vi "Img_PreProcess.vi"(4 "copy_name":string="untitled", 6 "copy_img":bool, 8 "error in (no error)":errorcluster, 11 "Original Img":T1) -> (0 "error out":errorcluster, 2 "transformed_out":T1, 3 "Original Img out":T1)   [LabVIEW 2021, in "Framework_lib.lvlib"]
uses:
  QMH/Framework_lib.lvlib
  <vilib>/vision/Image Controls.llb/IMAQ Image.ctl
  <vilib>/vision/NI_Vision_Development_Module.lvlib
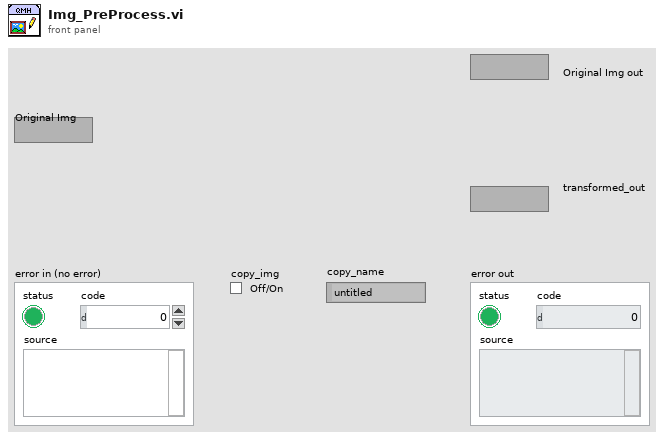
[diagram p1: front panel]
types:
  T1 = typedef "IMAQ Image.ctl" = refnum<image>
  T2 = cluster{"Brightness":sgl, "Contrast":sgl, "Gamma":sgl}
  T3 = typedef "Image Type" = u32
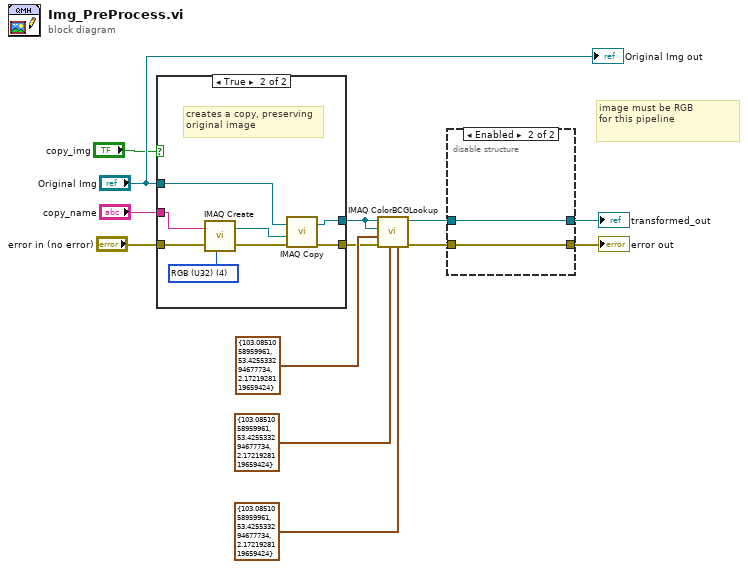
[diagram p0: block diagram]
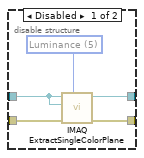
[diagram p2: hidden frame]
diagram:
  # "image must be RGB\nfor this pipeline"
  n1 = case shown="True" "copy_img" {
    tunnel: "error in (no error)" -> [w15 w23]
    tunnel: [w15 w22] -> w6
    tunnel: "Original Img" -> [w14 w21]
    tunnel: [w14 w20] -> w1
    tunnel: "copy_name" -> [_ w18]
    frame False {
      # "will transform orignial image"
    }
    frame True {
      w17 = T3 4 items=["Grayscale (U8)", "Grayscale (I16)", "Grayscale (SGL)", "Complex (CSG)", "RGB (U32)", "HSL (U32)", "RGB (U64)", "Grayscale (U16)"] ("Image Type")
      # "creates a copy, preserving\noriginal image"
      n2 = call "IMAQ Create"("Image Name"=w18, "Image Type"=w17, "error in (no error)"=w23) -> ("New Image"=w16:T1, "error out"=w19:errorcluster)  [unwired: 2 in]
      n3 = call "IMAQ Copy"("error in (no error)"=w19, "Image Dst"=w16, "Image Src"=w21) -> ("error out"=w22:errorcluster, "Image Dst Out"=w20:T1)  [unwired: 3 in]
    }
  }
  n4 = call "IMAQ ColorBCGLookup"("Blue BCG Values"=T2 {"Brightness"=103.085106, "Contrast"=53.425533, "Gamma"=2.1721928}, "Green BCG Values"=T2 {"Brightness"=103.085106, "Contrast"=53.425533, "Gamma"=2.1721928}, "error in (no error)"=w6, "Red BCG Values"=T2 {"Brightness"=103.085106, "Contrast"=53.425533, "Gamma"=2.1721928}, "Image Dst"=w1, "Image Src"=w1) -> ("error out"=w8:errorcluster, "Image Dst Out"=w3:T1)  [unwired: 1 in, 3 out]
  n5 = disable-structure shown="Enabled" {
    disable-tunnel: [w28 w29] -> w13
    disable-tunnel: [w27 w30] -> w12
    disable-tunnel: w8 -> [w25 w30]
    disable-tunnel: w3 -> [w24 w29]
    frame Disabled {
      w26 = 5 items=["Red", "Green", "Blue", "Hue", "Saturation", "Luminance", "Value", "Intensity"] ("Color Plane")
      n6 = call "IMAQ ExtractSingleColorPlane"("Color Plane"=w26, "error in (no error)"=w25, "Image Dst"=w24, "Image Src"=w24) -> ("error out"=w27:errorcluster, "Image Dst Out"=w28:T1)  [unwired: 6 out]
    }
    frame Enabled {
    }
  }
  "transformed_out" <- w13
  "error out" <- w12
  "Original Img out" <- "Original Img"
